vi "Remove Process from Map.vi"(8 "error in (no error)":errorcluster, 10 "Process Name":string, 11 "Application in":refnum<class "Application.lvclass">) -> (0 "error out":errorcluster, 2 "Process":refnum<class "Process.lvclass">, 3 "Application out":refnum<class "Application.lvclass">)   [LabVIEW 2020, in "Application.lvclass"]
uses:
  Application.lvclass
  <vilib>/Utility/error.llb/Error Cluster From Error Code.vi
  <vilib>/ErrorRing/Error Ring.xnode
  Process/Process.lvclass
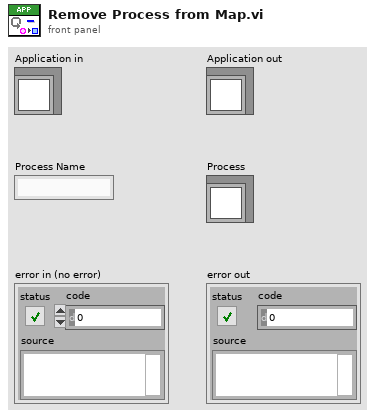
[diagram p1: front panel]
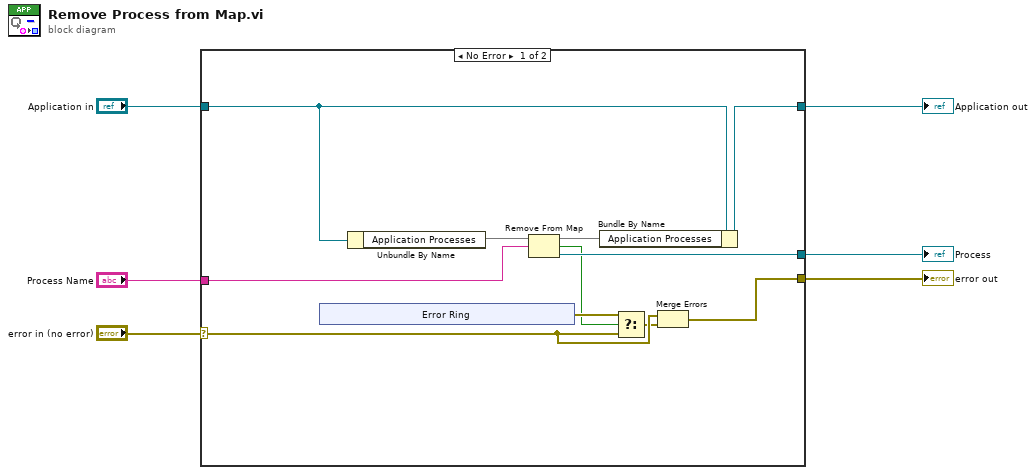
[diagram p0: block diagram]
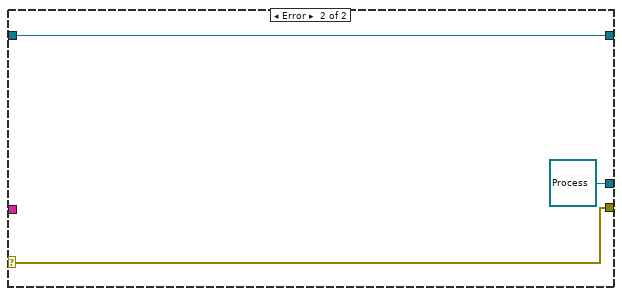
[diagram p2: hidden frame]
diagram:
  n1 = case shown="No Error" "error in (no error)" {
    selector: "error in (no error)" -> [w12 w24]
    tunnel: [w17 refnum<class "Process.lvclass"> refnum ("Process")] -> w6
    tunnel: [w16 w24] -> w5
    tunnel: [w15 w23] -> w4
    tunnel: "Application in" -> [w13 w23]
    tunnel: "Process Name" -> [w9 _]
    frame No Error {
      n2 = xnode "Error Ring"() -> ("error out"=w10:errorcluster)
      n3 = Unbundle By Name(w13) -> ("Application Processes"=w7:map{string, refnum<class "Process.lvclass">})
      n4 = Remove From Map(10:w9, 11:w7) -> (1:w17:refnum<class "Process.lvclass">, 2:w8:bool, 3:w14:map{string, refnum<class "Process.lvclass">})
      n5 = Bundle By Name(cluster=w13, "Application Processes"=w14) -> (w15:refnum<class "Application.lvclass">)
      n6 = Select(t=w10, s=w8, f=w12) -> (s? t:f=w11:errorcluster)
      n7 = Merge Errors(w12, w11) -> (w16:errorcluster)
    }
    frame Error {
    }
  }
  "Process" <- w6
  "error out" <- w5
  "Application out" <- w4
